vi "SetRunProgram.vi"(6 "Single step mode? (F)":bool, 7 "Resume from Stop? (F)":bool, 8 "error in (no error)":errorcluster, 9 "Starting interval number":u16=1 min=1 max=300 step=1, 10 "8800 Program Name (without .pgm extension)":string="test", 11 "VISA resource name":refnum<visa-resource-name>) -> (0 "error out":errorcluster, 3 "VISA resource name out":refnum<visa-resource-name>)   [LabVIEW 2023, in "Thermotron 8800.lvlib"]
doc: "RUNP\nCommand name: Run program mode\nCommand type: Control\nDescription: Places a stopped 8800 in run program mode, and specifies the program and starting interval.\nSyntax: RUNPp,I,R[,S]\nWhere:\np Program name (NOTE: The program must be in the root directory of the 8800’s hard drive.)\ni Interval number\nR Resume from stop\nS Single-step mode. This places the program in hold program mode at the end of each interval. To continue executing the program, send the RESM command.\nData type: See Syntax.\nOperation example: RUNPsimple_test,5,S\n8800 response: The 8800 runs program simple_test.pgm, starting at interval 5, in single-step mode."
uses:
  Thermotron 8800.lvlib
panel:
  out "8800 response":string
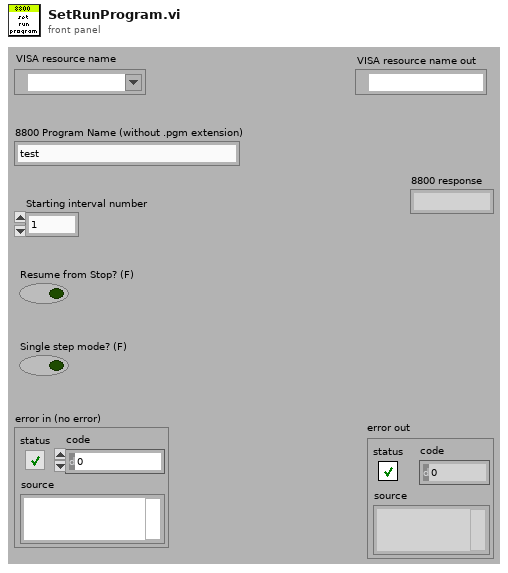
[diagram p1: front panel]
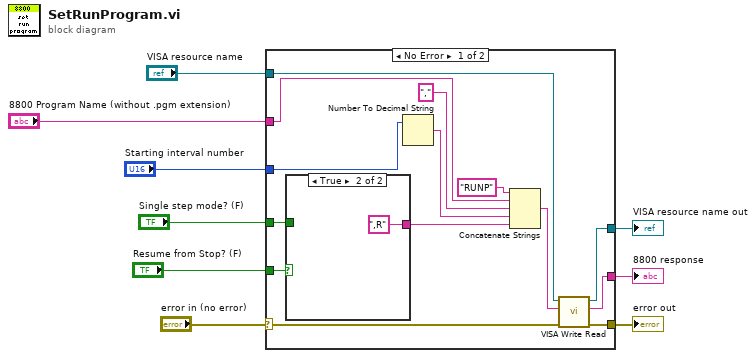
[diagram p0: block diagram]
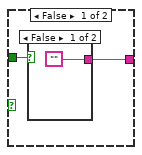
[diagram p2: hidden frame]
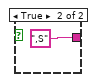
[diagram p3: hidden frame]
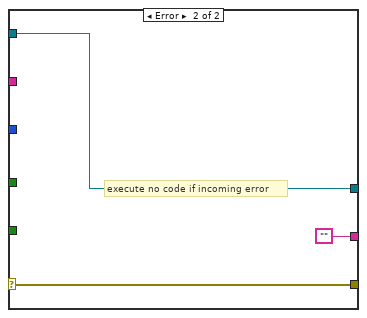
[diagram p4: hidden frame]
diagram:
  n1 = case shown="No Error" "error in (no error)" {
    selector: "error in (no error)" -> [w10 w31]
    tunnel: "VISA resource name" -> [w23 w30]
    tunnel: [w22 w30] -> w7
    tunnel: [w21 w31] -> w8
    tunnel: "8800 Program Name (without .pgm extension)" -> [w19 _]
    tunnel: "Starting interval number" -> [w17 _]
    tunnel: "Resume from Stop? (F)" -> [w15 _]
    tunnel: "Single step mode? (F)" -> [w13 _]
    tunnel: [w11 "" ("read buffer")] -> w2
    frame No Error {
      n2 = case shown="True" w15 {
        tunnel: [w24 ",R" ("8800 Command")] -> w14
        tunnel: w13 -> [w25 _]
        frame False {
          n3 = case shown="False" w25 {
            tunnel: ["" ",S" ("8800 Command")] -> w24
            frame False {
            }
            frame True {
            }
          }
        }
        frame True {
        }
      }
      n4 = Number To Decimal String(number=w17) -> (decimal integer string=w16:string)  [unwired: 1 in]
      n5 = Concatenate Strings("RUNP" ("8800 Command"), w19, "," ("8800 Command"), w16, w14) -> (w12:string)
      n6 = call "VISA Write Read.vi"("error in (no error)"=w10, "8800 Command"=w12, "VISA Refnum in"=w23) -> ("error out"=w21:errorcluster, "read buffer"=w11:string, "VISA Refnum out"=w22:refnum<visa-resource-name>)  [unwired: 6 in]
    }
    frame Error {
      # "execute no code if incoming error"
    }
  }
  "VISA resource name out" <- w7
  "error out" <- w8
  "8800 response" <- w2
